vi "Read Items.vi"(8 "error in (no error)":errorcluster, 11 "Selector in":refnum<class "Selector.lvclass">) -> (0 "error out":errorcluster, 2 "Items":T1(array[cluster]), 3 "Selector out":refnum<class "Selector.lvclass">)   [LabVIEW 2019, in "Selector.lvclass"]
uses:
  Selector.lvclass
  Selector.lvclass/Selector.ctl
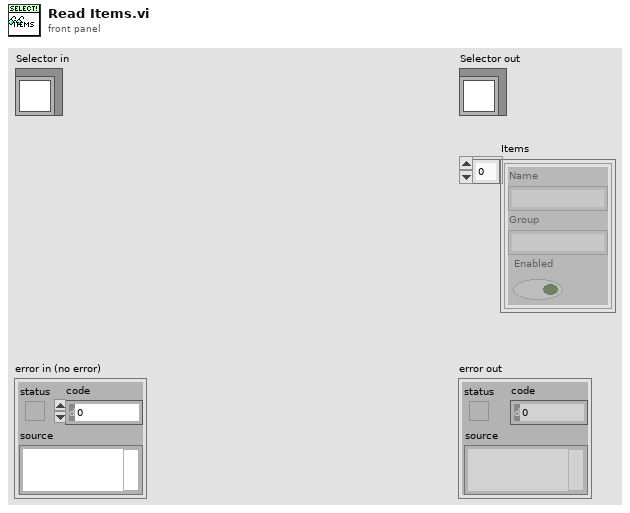
[diagram p1: front panel]
types:
  T1 = cluster{"Name":string, "Group":string, "Enabled":bool}[]
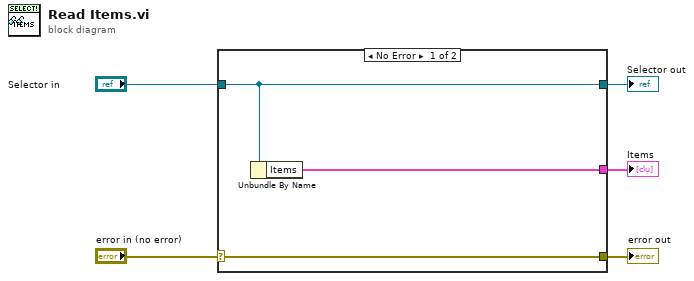
[diagram p0: block diagram]
diagram:
  n1 = case shown="No Error" "error in (no error)" {
    selector: "error in (no error)" -> [w8 w9]
    tunnel: [w8 w9] -> w4
    tunnel: [w7 w10] -> w2
    tunnel: "Selector in" -> [w7 w10]
    tunnel: [w6 _] -> w1
    frame No Error {
      n2 = Unbundle By Name(w7) -> ("Items"=w6:T1)
    }
    frame Error {
    }
  }
  "error out" <- w4
  "Selector out" <- w2
  "Items" <- w1
